vi "Read Relays.vi"(8 "error in (no error)":errorcluster, 11 "Switch Action Processor in":refnum<class "Switch Action Processor.lvclass">) -> (0 "error out":errorcluster, 2 "Relays":refnum<class "Relay.lvclass">[](array[class]), 3 "Switch Action Processor out":refnum<class "Switch Action Processor.lvclass">)   [LabVIEW 2016, in "SLSC Switch.lvlib" / "Switch Action Processor.lvclass"]
uses:
  Switch Action Processor.lvclass
  Relay/Relay.lvclass
  Switch Action Processor.lvclass/Switch Action Processor.ctl
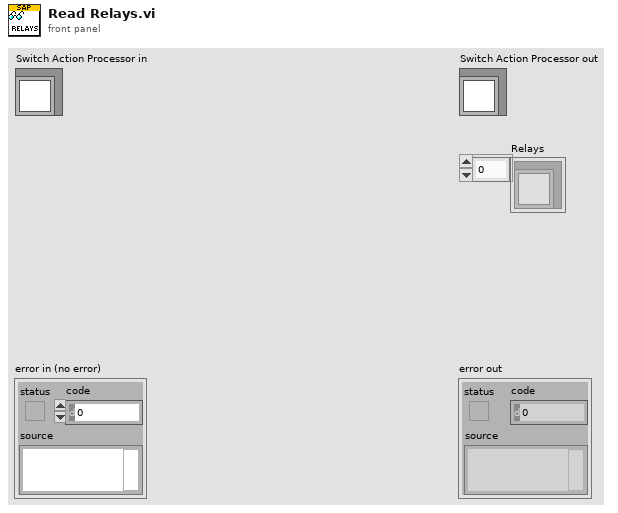
[diagram p1: front panel]
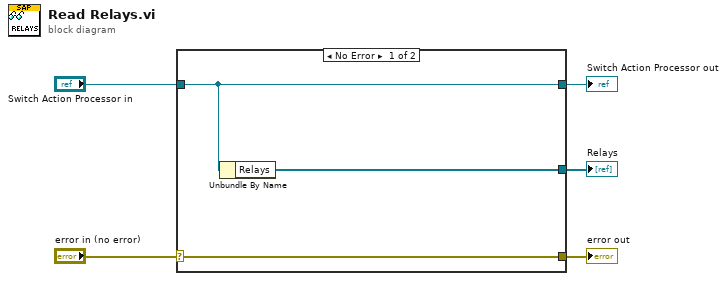
[diagram p0: block diagram]
diagram:
  n1 = case shown="No Error" "error in (no error)" {
    selector: "error in (no error)" -> [w8 w9]
    tunnel: [w8 w9] -> w4
    tunnel: [w7 w10] -> w2
    tunnel: "Switch Action Processor in" -> [w7 w10]
    tunnel: [w6 _] -> w1
    frame No Error {
      n2 = Unbundle By Name(w7) -> ("Relays"=w6:refnum<class "Relay.lvclass">[])
    }
    frame Error {
    }
  }
  "error out" <- w4
  "Switch Action Processor out" <- w2
  "Relays" <- w1
